vi "Write Filtered Errors.vi"(8 "error in (no error)":errorcluster, 10 "Filtered Errors":set{i32}(c389), 11 "Error Manager in":refnum<class "Error Manager.lvclass">) -> (0 "error out":errorcluster, 3 "Error Manager out":refnum<class "Error Manager.lvclass">)   [LabVIEW 2026, in "TALOS.lvlib" / "Error Manager.lvlib" / "Error Manager.lvclass"]
uses:
  Error Manager.lvclass
  Error Manager.lvclass/Error Manager.ctl
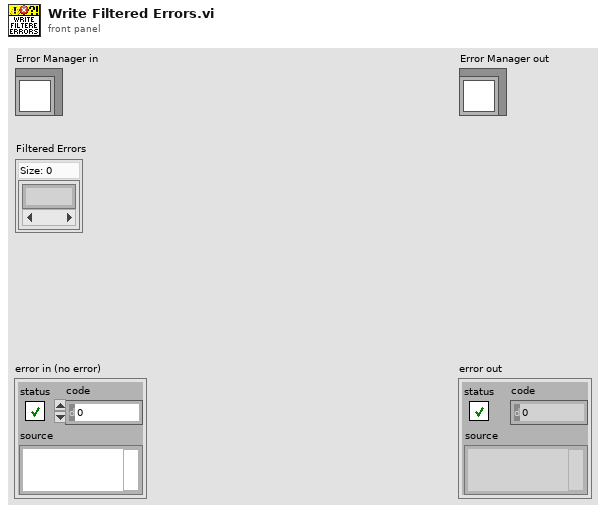
[diagram p1: front panel]
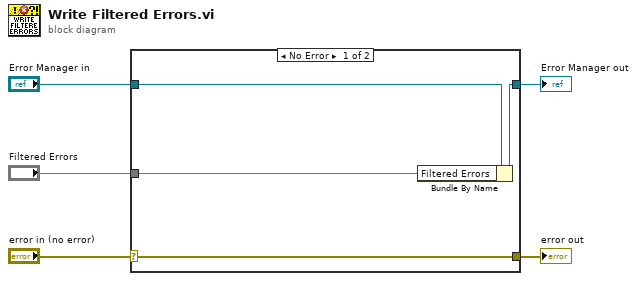
[diagram p0: block diagram]
diagram:
  n1 = case shown="No Error" "error in (no error)" {
    selector: "error in (no error)" -> [w9 w10]
    tunnel: [w9 w10] -> w4
    tunnel: [w7 w11] -> w2
    tunnel: "Error Manager in" -> [w8 w11]
    tunnel: "Filtered Errors" -> [w6 _]
    frame No Error {
      n2 = Bundle By Name(cluster=w8, "Filtered Errors"=w6) -> (w7:refnum<class "Error Manager.lvclass">)
    }
    frame Error {
    }
  }
  "error out" <- w4
  "Error Manager out" <- w2
